vi "Calc Mean.vi"(11 "JSON Statistics in":refnum<class "JSON Running Mean.lvclass">) -> (3 "JSON Value":refnum<class "JSON Value.lvclass">)   [LabVIEW 2020, in "Library Commun.lvlib" / "JSON Running Mean.lvclass"]
uses:
  JSON Running Mean.lvclass
  JSON Value/JSON Value.lvclass
  JSON Running Mean.lvclass/JSON Running Mean.ctl
  JSON Scalar/JSON Scalar.lvclass
  C:/Users/ngarcin/OneDrive - Altyor/Standard TB/Class/JSON API/JSON Value/JSON Value.lvclass
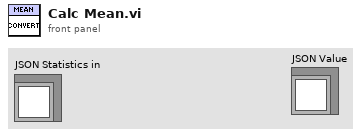
[diagram p1: front panel]
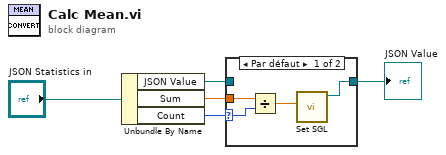
[diagram p0: block diagram]
diagram:
  n1 = Unbundle By Name("JSON Statistics in") -> ("JSON Value"=w4:refnum<class "JSON Value.lvclass">, "Sum"=w1:sgl, "Count"=w2:i32)
  n2 = case shown="Par défaut" w2 {
    selector: w2 -> [w7 _]
    tunnel: [w9 w10] -> w3
    tunnel: w4 -> [_ w10]
    tunnel: w1 -> [w8 _]
    frame Default {
      n3 = Divide(x=w8, y=w7) -> (x/y=w6:sgl)
      n4 = call "Set SGL.vi"("Numeric"=w6) -> ("JSON Scalar out"=w9:refnum<class "JSON Scalar.lvclass">)  [unwired: 9 in, 1 out]
    }
    frame ..0 {
    }
  }
  "JSON Value" <- w3
